vi "Time for ERD Value Change.vi"(0 "GEA2 Reference In":refnum<k24>, 1 "GEA Inputs":T3 {"Destination" format="%.0x"; "Source" format="%.0x"}, 2 "Standalone?":bool, 3 "Read ERD List":T1 {"ERD Number" format="%.0x"}, 5 "Upper Limit":dbl, 7 "Expected Time":dbl, 9 "Lower Limit":dbl, 11 "Error In":errorcluster, 12 "Expected ERD Response":string, 13 "Equal?":bool) -> (4 "GEA2 Reference Out":refnum<k24>, 6 "Pass/Fail?":bool, 10 "Report Text":string, 15 "Error Out":errorcluster)   [LabVIEW 2016, in "TL27.lvlib"]
doc: "This vi can be used to read ERD every 1 sec for user selected repeat counts."
uses:
  Projects/TL27.lvlib
  C:/Automation/DLLs/PC Dot Net/GeaCommunication.dll
  Common/LabVIEW GEA2 Toolkit/LabVIEW_GEA2_Toolkit.lvlibp/type defs/Source_Destination.ctl
  Common/LabVIEW GEA2 Toolkit/LabVIEW_GEA2_Toolkit.lvlibp/type defs/ERD Read Data In.ctl
  Common/LabVIEW GEA2 Toolkit/LabVIEW_GEA2_Toolkit.lvlibp/type defs/Data Type.ctl
  Common/LabVIEW GEA2 Toolkit/LabVIEW_GEA2_Toolkit.lvlibp
panel:
  out "Data":string
  out "x-y":dbl
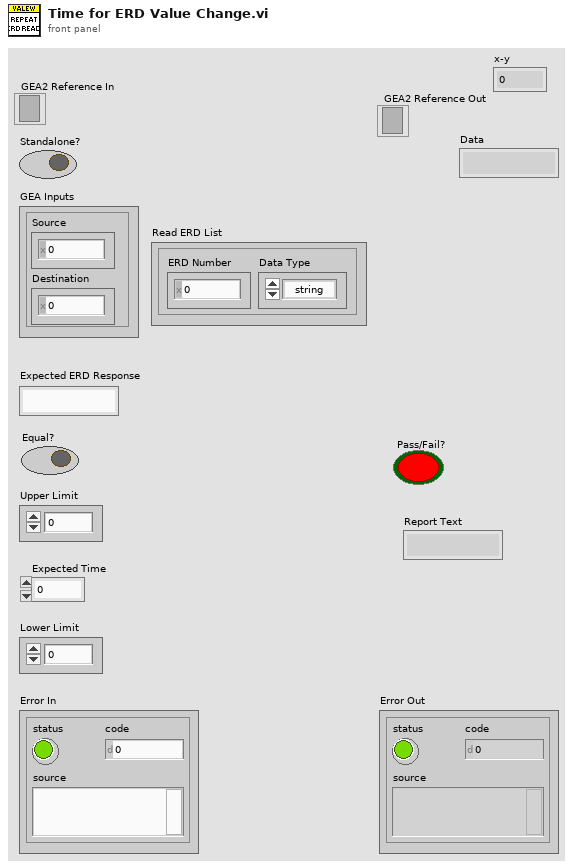
[diagram p1: front panel]
types:
  T1 = typedef "LabVIEW_GEA2_Toolkit.lvlibp/ERD Read Data In.ctl" = cluster{"ERD Number":u16, "Data Type":T2}
  T2 = typedef "LabVIEW_GEA2_Toolkit.lvlibp/Data Type.ctl" = enum16{"string", "boolean", "uint8_t", "uint16_t", "uint32_t", "uint64_t", "int8_t", "int16_t", "int32_t", "int64_t"}
  T3 = typedef "LabVIEW_GEA2_Toolkit.lvlibp/Source_Destination.ctl" = cluster{"Source":u8, "Destination":u8}
  T4 = typedef "LabVIEW_GEA2_Toolkit.lvlibp/ERD Read Data Out.ctl" = cluster{"ERD Number":u16, "Data":string}
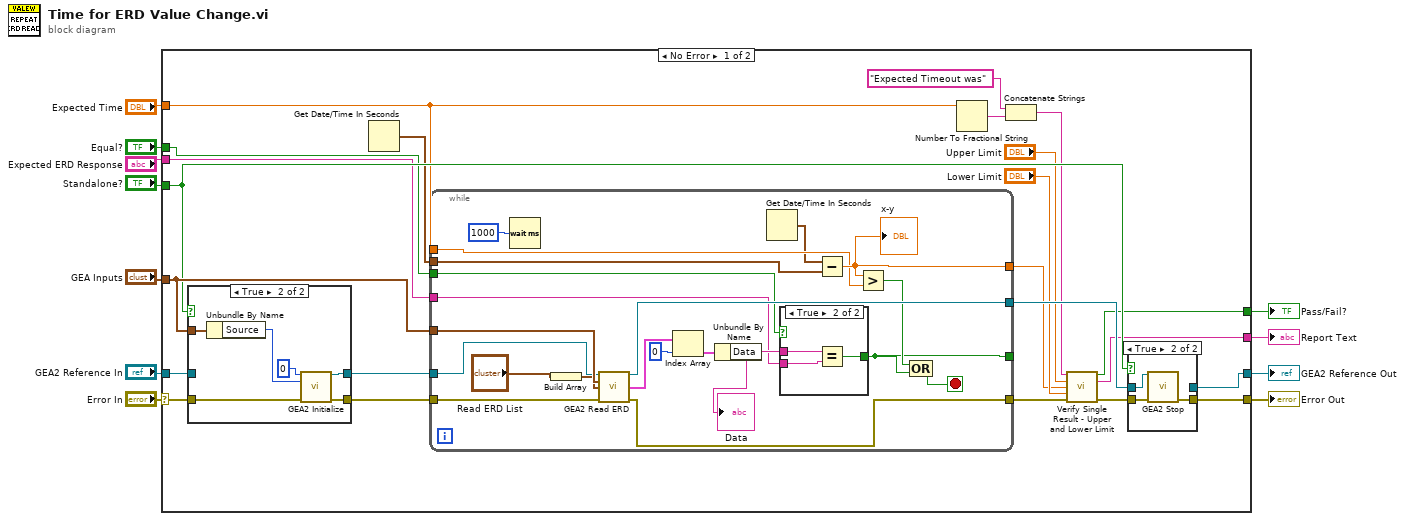
[diagram p0: block diagram]
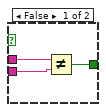
[diagram p2: hidden frame]
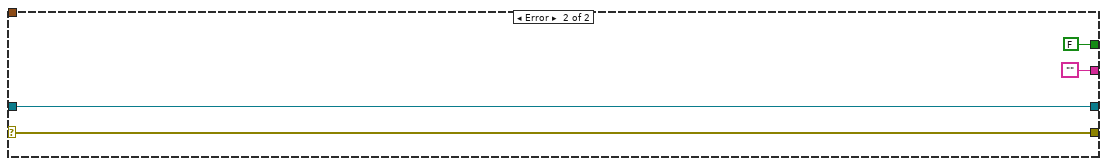
[diagram p5: hidden frame]
diagram:
  n1 = case shown="No Error" "Error In" {
    selector: "Error In" -> [w12 w75]
    tunnel: "GEA Inputs" -> [w34 _]
    tunnel: [w33 w75] -> w10
    tunnel: "GEA2 Reference In" -> [w32 w78]
    tunnel: "Standalone?" -> [w31 _]
    tunnel: [w29 w78] -> w7
    tunnel: "Expected ERD Response" -> [w27 _]
    tunnel: "Equal?" -> [w26 _]
    tunnel: "Expected Time" -> [w20 _]
    tunnel: [w14 FALSE ("Pass/Fail?")] -> w3
    tunnel: [w13 ""] -> w2
    frame No Error {
      n2 = case shown="True" w31 {
        tunnel: w12 -> [w67 w74]
        tunnel: [w67 w73] -> w25
        tunnel: w32 -> [w68 _]
        tunnel: [w68 w72] -> w30
        tunnel: w34 -> [_ w70]
        frame False {
        }
        frame True {
          n3 = Unbundle By Name(w70) -> ("Source"=w71:u8)
          n4 = call "GEA2 Initialize.vi"("Board Index"=0, "Source Address"=w71, "error in"=w74) -> ("GEA2 Reference Out"=w72:refnum<k24>, "error out"=w73:errorcluster)  [unwired: 10 in, 1 out]
        }
      }
      n5 = Get Date/Time In Seconds() -> (seconds since 1Jan1904=w24:timestamp)
      n6 = while {
        tunnel: w34 -> [w55]
        tunnel: [w50] -> w16
        tunnel: [w54] -> w28
        tunnel: w30 -> [w53]
        tunnel: w25 -> [w52]
        tunnel: w27 -> [w45]
        tunnel: w26 -> [w44]
        tunnel: [w40] -> _
        tunnel: w24 -> [w35]
        tunnel: [w43] -> w21
        tunnel: w20 -> [w42]
        stop <- w39 stop-if-true
        n7 = Wait (ms)(milliseconds to wait=u32 1000) -> ()  [unwired: 1 out]
        n8 = Build Array("Read ERD List") -> (w38:T1[])
        n9 = call "GEA2 Read ERD.vi"("GEA2 Reference In"=w53, "GEA Inputs"=w55, "Read ERD List"=w38, "Error In"=w52) -> ("GEA2 Reference Out"=w54:refnum<k24>, "ERD Data Out"=w49:T4[], "Error Out"=w50:errorcluster)  [unwired: 8 in, 1 out]
        n10 = Index Array(array=w49, index=0) -> (element=w47:T4)
        n11 = Unbundle By Name(w47) -> ("Data"=w46:string)
        "Data" <- w46
        n12 = Get Date/Time In Seconds() -> (seconds since 1Jan1904=w36:timestamp)
        n13 = case shown="True" w44 {
          tunnel: w46 -> [w58 w61]
          tunnel: w45 -> [w57 w60]
          tunnel: [w56 w59] -> w40
          frame False {
            n14 = Not Equal?(x=w58, y=w57) -> (x != y?=w56:bool)
          }
          frame True {
            n15 = Equal?(x=w61, y=w60) -> (x = y?=w59:bool)
          }
        }
        n16 = Subtract(x=w36, y=w35) -> (x-y=w43:dbl)
        "x-y" <- w43
        n17 = Greater?(x=w43, y=w42) -> (0:w41:bool)
        n18 = Compound Arithmetic op=OR(w41, w40) -> (w39:bool)
      }
      n19 = Number To Fractional String(number=w20) -> (F-format string=w18:string)  [unwired: 3 in]
      n20 = Concatenate Strings("Expected Timeout was", w18) -> (w17:string)
      n21 = call "Verify Single Result - Upper and Lower Limit.vi"("Name"=w17, "Upper Limit"="Upper Limit", "Value"=w21, "Lower Limit"="Lower Limit", "Error In"=w16) -> ("Pass/Fail?"=w14:bool, "Report Text"=w13:string, "Error Out"=w15:errorcluster)  [unwired: 8 in]
      n22 = case shown="True" w31 {
        tunnel: w15 -> [w62 w65]
        tunnel: [w62 w64] -> w33
        tunnel: w28 -> [w63 w66]
        tunnel: [w63 _] -> w29
        frame False {
        }
        frame True {
          n23 = call "GEA2 Stop.vi"("GEA2 Reference In"=w66, "Error In"=w65) -> ("Error Out"=w64:errorcluster)  [unwired: 13 in]
        }
      }
    }
    frame Error {
    }
  }
  "Error Out" <- w10
  "GEA2 Reference Out" <- w7
  "Report Text" <- w2
  "Pass/Fail?" <- w3
